vi "GFITS_updateHeaders.vi"(0 "fref":u64, 1 "nodeID":string, 3 "Multiple extensions?":bool, 5 "num of extensions":u16=16, 6 "number of keywords":i32[](array[numeric]), 9 "expID in":string, 11 "error in (no error)":errorcluster, 12 "Database RefNum in":T1, 13 "headers":bool=TRUE) -> (4 "ref out":u64, 10 "expID":string, 15 "error out":errorcluster)   [LabVIEW 2016]
uses:
  DBSHAND/private/vis/DatabaseHand_RefNum.ctl
  Common/public/vis/CMN_FVAR_action.ctl
  GFITS_Gbls.vi
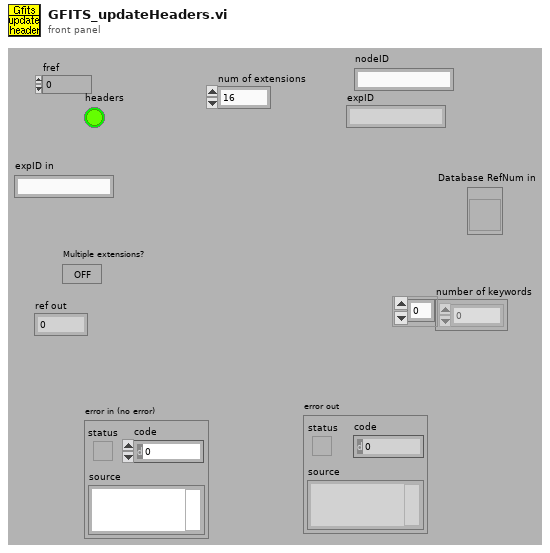
[diagram p1: front panel]
types:
  T1 = typedef "DatabaseHand_RefNum.ctl" = refnum<vi>
  T2 = enum16{"clear all", "add extension", "add keyword", "get", "clear extension", "done"}
  T3 = typedef "CMN_FVAR_action.ctl" = enum16{"read", "write"}
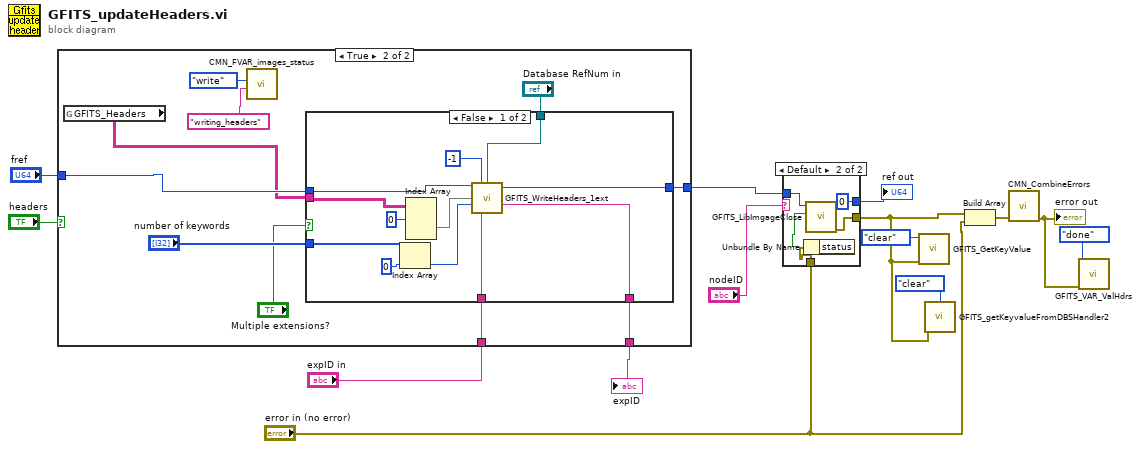
[diagram p0: block diagram]
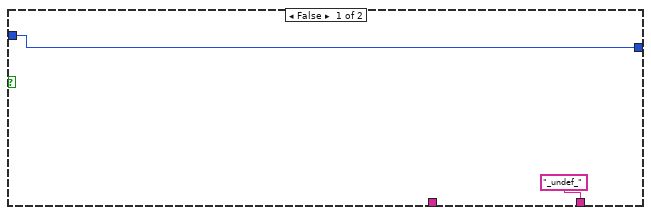
[diagram p2: hidden frame]
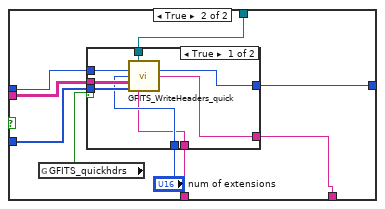
[diagram p3: hidden frame]
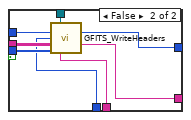
[diagram p4: hidden frame]
diagram:
  n1 = case shown="True" "headers" {
    tunnel: [w16 w26] -> w12
    tunnel: "fref" -> [w16 w25]
    tunnel: ["_undef_" ("expID") w20] -> w8
    tunnel: "expID in" -> [_ w17]
    frame False {
    }
    frame True {
      n2 = global read "GFITS_Gbls.vi" "GFITS_Headers"() -> (w22:string[][][])
      n3 = call "CMN_FVAR_images_status.vi"("value in"="writing_headers", "action"=CMN_FVAR_action."write") -> ()  [unwired: 9 out]
      n4 = case shown="False" "Multiple extensions?" {
        tunnel: w25 -> [w38 w47]
        tunnel: [w31 w46] -> w26
        tunnel: w22 -> [w37 w45]
        tunnel: "number of keywords" -> [w34 w44]
        tunnel: "Database RefNum in" -> [w29 w43]
        tunnel: [w28 w40] -> w20
        tunnel: w17 -> [w27 w39]
        frame False {
          n5 = Index Array(array=w34, index=0 ("Index")) -> (element=w32:i32)
          n6 = Index Array(array=w37, index (dim 0)=0 ("Index (page)")) -> (element=w35:string[][])  [unwired: 2 in]
          n7 = call "GFITS_WriteHeaders_1ext.vi"("ref"=w38, "extension"=-1, "Database RefNum in"=w29, "Keywords"=w35, "numer of keywords"=w32, "expID in"=w27) -> ("ref out"=w31:u64, "expID"=w28:string)  [unwired: 1 in, 7 out]
        }
        frame True {
          n8 = global read "GFITS_Gbls.vi" "GFITS_quickhdrs"() -> (w42:bool)
          n9 = case shown="True" w42 {
            tunnel: w47 -> [w55 w63]
            tunnel: [w54 w62] -> w46
            tunnel: w45 -> [w53 w61]
            tunnel: w44 -> [w52 w60]
            tunnel: w43 -> [w51 w59]
            tunnel: "num of extensions" -> [w50 w58]
            tunnel: [w49 w57] -> w40
            tunnel: w39 -> [w48 w56]
            frame True {
              n10 = call "GFITS_WriteHeaders_quick.vi"("Database RefNum in"=w51, "ref"=w55, "number of extensions"=w50, "Keywords"=w53, "number of keywords"=w52, "expID in"=w48) -> ("ref out"=w54:u64, "expID"=w49:string)  [unwired: 8 out]
            }
            frame False {
              n11 = call "GFITS_WriteHeaders.vi"("Database RefNum in"=w59, "ref"=w63, "number of extensions"=w58, "Keywords"=w61, "number of keywords"=w60, "expID in"=w56) -> ("ref out"=w62:u64, "expID"=w57:string)  [unwired: 8 out]
            }
          }
        }
      }
    }
  }
  "expID" <- w8
  n12 = case shown="Default" "nodeID" {
    tunnel: [w65 u64 0 ("ref out")] -> w14
    tunnel: w12 -> [w65 w70]
    tunnel: [w64 w69] -> w6
    tunnel: "error in (no error)" -> [w64 w67]
    frame "MASTER" {
    }
    frame Default {
      n13 = Unbundle By Name(w67) -> ("status"=w66:bool)
      n14 = call "GFITS_LibImgageClose.vi"("err in"=w66, "fd"=w70) -> ("error out"=w69:errorcluster)  [unwired: 1 in, 8 out]
    }
  }
  "ref out" <- w14
  n15 = call "GFITS_GetKeyValue.vi"("error in (no error)"=w6, "action"=enum16{"get", "clear"}."clear") -> ()  [unwired: 1 in, 9 out]
  n16 = call "GFITS_getKeyvalueFromDBSHandler2.vi"("action"=enum16{"get", "clear"}."clear", "error in (no error)"=w6) -> ()  [unwired: 7 in, 7 out]
  n17 = Build Array(w6, "error in (no error)") -> (w5:errorcluster[])
  n18 = call "CMN_CombineErrors.vi"("Errors"=w5) -> ("error out"=w1:errorcluster)  [unwired: 10 out]
  "error out" <- w1
  n19 = call "GFITS_VAR_ValHdrs.vi"("action"=T2."done", "error in (no error)"=w1) -> ()  [unwired: 3 in, 11 out]
